vi "Keithley 2002 DCI Config.vi"(0 "GPIB address":string="16", 1 "integration time (0:auto)":u16(ring) items=["automatic", "automatic once", "set to minimum", "set to maximum", "set aperature value", "set NPLC value"], 2 "integ. value":dbl=0.01667 format="%^.2e", 3 "range (auto:0)":u16(ring) items=["autorange", "autorange once", "set min range", "set max range", "set range value"], 4 "range value (amps)":dbl=2.0 min=0.0002 max=2.0 format="%^.2e", 5 "error in":T1, 6 "method":bool=TRUE, 7 "resolution (4.5 digits:3)":u16(ring)=3 items=["auto resolution", "auto resolution once", "3.5 digits", "4.5 digits", "5.5 digits", "6.5 digits", "7.5 digits", "8.5 digits"], 8 "reference (off:0)":u16(ring) items=["off", "set reference value"], 9 "digital filter (off:0)":u16(ring) items=["off", "auto filter", "auto filter once", "moving filter", "repeating filter"], 10 "reference value (amps)":dbl min=-2.1 max=2.1 format="%^.2e", 11 "dig. filter count":dbl=10.0 min=1.0 max=100.0 step=1.0 format="%^.2e", 14 "advanced filter (off:0)":u16(ring) items=["off", "enabled"], 15 "noise tolerance (%)":dbl=1.0 min=0.0 max=100.0 step=1.0 format="%^.2e") -> (19 "error out":T1)   [LabVIEW 2020]
doc: "This VI is used to configure the settings for the DC current measurements. The instrument can be in any mode when this VI is run. The settings will go into effect and the instrument will go into the DC current mode."
panel:
  # "normal\nin-circuit"
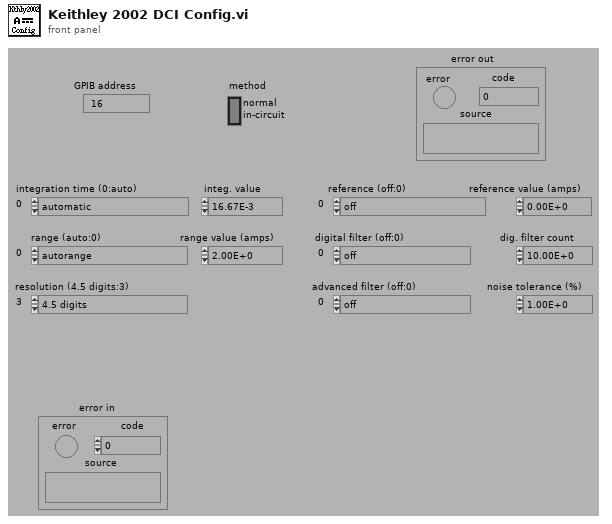
[diagram p1: front panel]
types:
  T1 = cluster{"error":bool, "code":i32, "source":string}
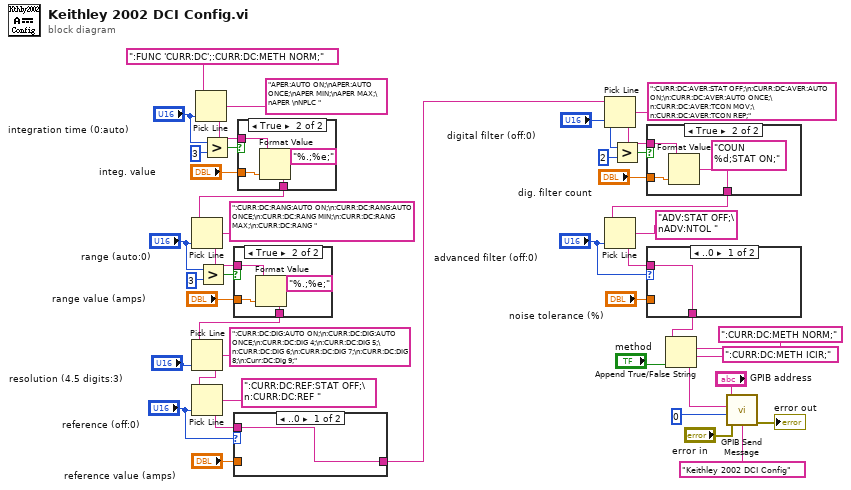
[diagram p0: block diagram]
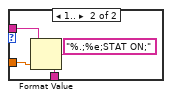
[diagram p2: hidden frame]
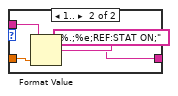
[diagram p4: hidden frame]
diagram:
  n1 = Pick Line(string ("")=":FUNC 'CURR:DC';:CURR:DC:METH NORM;", multi-line string="APER:AUTO ON;\nAPER:AUTO ONCE;\nAPER MIN;\nAPER MAX;\nAPER \nNPLC ", line index="integration time (0:auto)") -> (output string=w39:string)
  n2 = Greater?(x="range (auto:0)", y=3) -> (0:w37:bool)
  n3 = Greater?(x="integration time (0:auto)", y=3) -> (0:w40:bool)
  n4 = case shown="True" w40 {
    tunnel: "integ. value" -> [_ w48]
    tunnel: w39 -> [w45 w47]
    tunnel: [w45 w46] -> w1
    frame False {
    }
    frame True {
      n5 = Format Value(string ("")=w47, format string="%.;%e;", value (0)=w48) -> (output string=w46:string)
    }
  }
  n6 = Pick Line(string ("")=w1, multi-line string=":CURR:DC:RANG:AUTO ON;\n:CURR:DC:RANG:AUTO ONCE;\n:CURR:DC:RANG MIN;\n:CURR:DC:RANG MAX;\n:CURR:DC:RANG ", line index="range (auto:0)") -> (output string=w38:string)
  n7 = case shown="True" w37 {
    tunnel: "range value (amps)" -> [_ w53]
    tunnel: w38 -> [w50 w52]
    tunnel: [w50 w51] -> w30
    frame False {
    }
    frame True {
      n8 = Format Value(string ("")=w52, format string="%.;%e;", value (0)=w53) -> (output string=w51:string)
    }
  }
  n9 = Pick Line(string ("")=w30, multi-line string=":CURR:DC:DIG:AUTO ON;\n:CURR:DC:DIG:AUTO ONCE;\n:CURR:DC:DIG 4;\n:CURR:DC:DIG 5;\n:CURR:DC:DIG 6;\n:CURR:DC:DIG 7;\n:CURR:DC:DIG 8;\n:Curr:DC:Dig 9;", line index="resolution (4.5 digits:3)") -> (output string=w26:string)
  n10 = Pick Line(string ("")=w26, multi-line string=":CURR:DC:REF:STAT OFF;\n:CURR:DC:REF ", line index="reference (off:0)") -> (output string=w29:string)
  n11 = case shown="..0" "reference (off:0)" {
    tunnel: "reference value (amps)" -> [_ w59]
    tunnel: w29 -> [w55 w58]
    tunnel: [w55 w56] -> w5
    frame ..0 {
    }
    frame 1.. {
      n12 = Format Value(string ("")=w58, format string="%.;%e;REF:STAT ON;", value (0)=w59) -> (output string=w56:string)
    }
  }
  n13 = Pick Line(string ("")=w5, multi-line string=":CURR:DC:AVER:STAT OFF;\n:CURR:DC:AVER:AUTO ON;\n:CURR:DC:AVER:AUTO ONCE;\n:CURR:DC:AVER:TCON MOV;\n:CURR:DC:AVER:TCON REP;", line index="digital filter (off:0)") -> (output string=w23:string)
  n14 = Greater?(x="digital filter (off:0)", y=2) -> (0:w20:bool)
  n15 = case shown="True" w20 {
    tunnel: "dig. filter count" -> [_ w64]
    tunnel: w23 -> [w60 w63]
    tunnel: [w60 w62] -> w13
    frame False {
    }
    frame True {
      n16 = Format Value(string ("")=w63, format string="COUN %d;STAT ON;", value (0)=w64) -> (output string=w62:string)
    }
  }
  n17 = Pick Line(string ("")=w13, multi-line string="ADV:STAT OFF;\nADV:NTOL ", line index="advanced filter (off:0)") -> (output string=w16:string)
  n18 = case shown="..0" "advanced filter (off:0)" {
    tunnel: "noise tolerance (%)" -> [_ w69]
    tunnel: w16 -> [w65 w68]
    tunnel: [w65 w67] -> w4
    frame ..0 {
    }
    frame 1.. {
      n19 = Format Value(string ("")=w68, format string="%.;%e;STAT ON;", value (0)=w69) -> (output string=w67:string)
    }
  }
  n20 = Append True/False String(1:"method", 2:":CURR:DC:METH ICIR;", 3:":CURR:DC:METH NORM;", 4:w4) -> (0:w3:string)
  n21 = call "GPIB Send Message.vi"("address string"="GPIB address", "write buffer"=w3, "source"="Keithley 2002 DCI Config", "write mode (set END:0)"=0, "error in"="error in") -> ("error out"=→"error out":T1)  [unwired: 2 in, 2 out]
